vi "Activate SlavesHW.vi"(8 "error in (no error)":errorcluster, 9 "has been deactivated?":bool[](array[boolean]), 10 "DGNrs":i32[](array[numeric]), 11 "BME_DG_System in":refnum<class "BME_DG_System.lvclass">) -> (0 "error out":errorcluster, 3 "BME_DG_System out":refnum<class "BME_DG_System.lvclass">)   [LabVIEW 2009, in "POLARIS BME DG.lvlib" / "BME_DG_System.lvclass"]
doc: "Activates all slave DGs or a group of them.\n\nIf you wire inputs DGNrs and \"has been deactivated?\" only the deactivated slaves will be reactivated. \n\n\n---------------\n\nauthor: Alexander Kessler, Helmholtz-Institut-Jena \nmaintainer: Alexander Kessler: alexander.kessler@uni-jena.de\n\n\nLicense Agreement for this software:\n\nCopyright (C)\nHelmholtz-Institut-Jena\nFröbelsteg 3\n07743 Jena\nGermany\n\nContact: alexander.kessler@uni-jena.de\n\nThis program is free software; you can redistribute it and/or modify it under the terms of the GNU General Public License as published by the Free Software Foundation; either version 2 of the license, or (at your option) any later version.\n\nThis program is distributed in the hope that it will be useful, but WITHOUT ANY WARRANTY; without even the implied warranty of MERCHANTABILITY or FITNESS FOR A PARTICULAR PURPOSE. See the GNU General License for more details (http://www.gnu.org)."
uses:
  BME_DG_System.lvclass
  BME_DG_System.lvclass/BME_DG_System.ctl
  BME_DG_Base/BME_DG_Base.lvclass
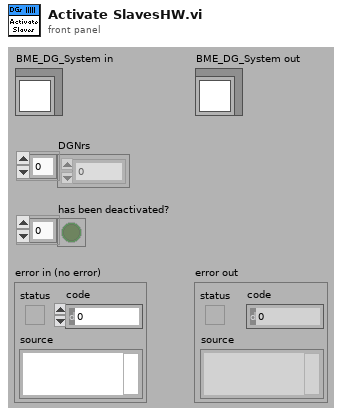
[diagram p1: front panel]
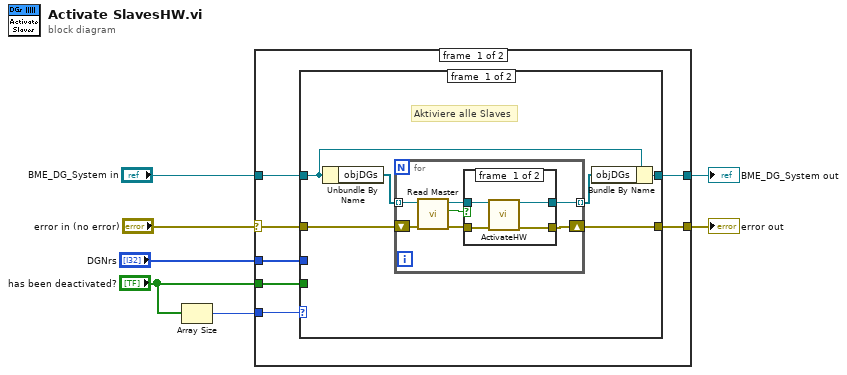
[diagram p0: block diagram]
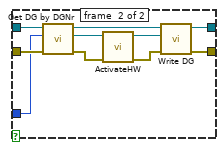
[diagram p4: hidden frame]
diagram:
  n1 = Array Size(array="has been deactivated?") -> (size(s)=w3:i32)
  n2 = case shown="No Error" "error in (no error)" {
    selector: "error in (no error)" -> [w13 w59]
    tunnel: [w11 w59] -> w6
    tunnel: [w12 w58] -> w4
    tunnel: "BME_DG_System in" -> [w14 w58]
    tunnel: w3 -> [w10 _]
    tunnel: "DGNrs" -> [w9 _]
    tunnel: "has been deactivated?" -> [w8 _]
    frame #0 {
      n3 = case shown="0" w10 {
        tunnel: w14 -> [w20 w37]
        tunnel: w13 -> [w18 w39]
        tunnel: [w17 w36] -> w12
        tunnel: [w15 w38] -> w11
        tunnel: w9 -> [_ w35]
        tunnel: w8 -> [_ w34]
        frame #0 {
          # "Aktiviere alle Slaves"
          n4 = Unbundle By Name(w20) -> ("objDGs"=w19:refnum<class "BME_DG_Base.lvclass">[])
          n5 = for {
            tunnel: w19 -> [w25] mode=indexing
            tunnel: [w26] -> w16 mode=indexing
            shift-right: [w27] -> w15
            shift-left: w18 -> [w21]
            n6 = call-dynamic "Read Master.vi"("error in (no error)"=w21, "BME_DG_Base in"=w25) -> ("error out"=w23:errorcluster, "Master?"=w22:bool, "BME_DG_Base out"=w24:refnum<class "BME_DG_Base.lvclass">)  [unwired: 6 in, 1 out]
            n7 = case shown="False" w22 {
              tunnel: w24 -> [w31 w33]
              tunnel: w23 -> [w30 w32]
              tunnel: [w29 w32] -> w27
              tunnel: [w28 w33] -> w26
              frame #0 {
                n8 = call "ActivateHW.vi"("error in (no error)"=w30, "BME_DG_Base in"=w31) -> ("error out"=w29:errorcluster, "BME_DG_Base out"=w28:refnum<class "BME_DG_Base.lvclass">)  [unwired: 8 in]
              }
              frame #1 {
              }
            }
          }
          n9 = Bundle By Name(cluster=w20, "objDGs"=w16) -> (w17:refnum<class "BME_DG_System.lvclass">)
        }
        frame #1 {
          # "Falls DGNrs und has been deactivated verdahtet sijnd\nAktiviere nur Karten, die vorher auch wirklich deaktivert\nwurden"
          n10 = for {
            shift-right: [w40] -> w38
            shift-left: w39 -> [w44]
            shift-right: [w41] -> w36
            shift-left: w37 -> [w45]
            tunnel: w35 -> [w43] mode=indexing
            tunnel: w34 -> [w42] mode=indexing
            n11 = case shown="True" w42 {
              tunnel: w45 -> [w47 w57]
              tunnel: w44 -> [w46 w56]
              tunnel: w43 -> [_ w55]
              tunnel: [w47 w49] -> w41
              tunnel: [w46 w48] -> w40
              frame #0 {
              }
              frame #1 {
                n12 = call "Get DG by DGNr.vi"("error in (no error)"=w56, "DG Nr."=w55, "BME_DG_System in"=w57) -> ("error out"=w53:errorcluster, "BME_DG_Base.lvclass"=w52:refnum<class "BME_DG_Base.lvclass">, "BME_DG_System out"=w54:refnum<class "BME_DG_System.lvclass">)  [unwired: 5 in, 1 out]
                n13 = call "ActivateHW.vi"("error in (no error)"=w53, "BME_DG_Base in"=w52) -> ("error out"=w50:errorcluster, "BME_DG_Base out"=w51:refnum<class "BME_DG_Base.lvclass">)  [unwired: 8 in]
                n14 = call "Write DG.vi"("error in (no error)"=w50, "BME_DG_Base"=w51, "BME_DG_System in"=w54) -> ("error out"=w48:errorcluster, "BME_DG_System out"=w49:refnum<class "BME_DG_System.lvclass">)  [unwired: 7 in]
              }
            }
          }
        }
      }
    }
    frame #1 {
    }
  }
  "error out" <- w6
  "BME_DG_System out" <- w4
